vi "GetGreyscalePlane.vi"(1 "Image In":T1 {"Dialogs" format="%.0b"}) -> (0 "Greyscale  Out":T1 {"Dialogs" format="%.0b"})   [LabVIEW 2024]
uses:
  <userlib>/ImageProcessing/QTLIB_2595_LV86/QT_Image.ctl
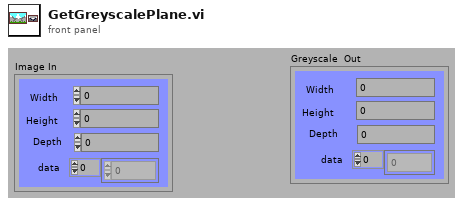
[diagram p1: front panel]
types:
  T1 = typedef "QT_Image.ctl" = cluster{"Width":i32, "Height":i32, "Depth":i32, "data":u8[], "Compressed data":u8[], "Color table":u32[], "Duration":i32, "Options":i32, "Timestamp":i32, "ID":i32, "Reserved":i32, "Dialogs":u32}
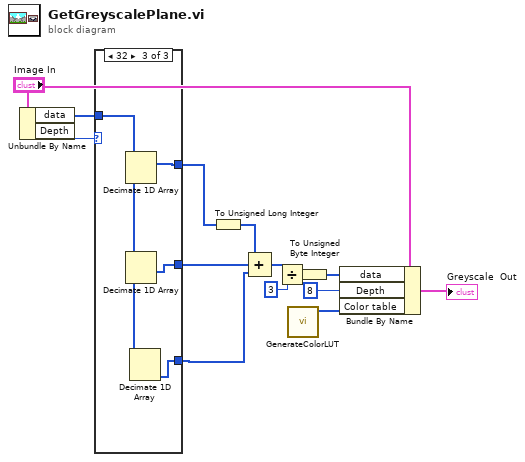
[diagram p0: block diagram]
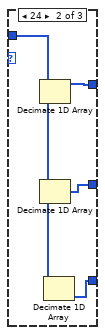
[diagram p3: hidden frame]
diagram:
  n1 = Unbundle By Name("Image In") -> ("data"=w14:u8[], "Depth"=w13:i32)
  n2 = case shown="32" w13 {
    tunnel: [w15 w17 w21] -> w12
    tunnel: w14 -> [w15 w19 w23]
    tunnel: [w15 w18 w22] -> w11
    tunnel: [w15 w16 w20] -> w10
    frame Default {
    }
    frame 24 {
      n3 = Decimate 1D Array(w19) -> (w17:u8[])  [unwired: 2 out]
      n4 = Decimate 1D Array(w19) -> (w18:u8[])  [unwired: 2 out]
      n5 = Decimate 1D Array(w19) -> (w16:u8[])  [unwired: 2 out]
    }
    frame 32 {
      n6 = Decimate 1D Array(w23) -> (w21:u8[])  [unwired: 3 out]
      n7 = Decimate 1D Array(w23) -> (w22:u8[])  [unwired: 3 out]
      n8 = Decimate 1D Array(w23) -> (w20:u8[])  [unwired: 3 out]
    }
  }
  n9 = To Unsigned Long Integer(number=w12) -> (unsigned 32bit integer=w9:u32[])
  n10 = Compound Arithmetic op=ADD(w9, w11, w10) -> (w8:u32[])
  n11 = Divide(x=w8, y=3 ("Depth")) -> (x/y=w5:dbl[])
  n12 = call <userlib>:"GenerateColorLUT.vi"() -> ("Greyscale"=w2:u32[])  [unwired: 4 out]
  n13 = To Unsigned Byte Integer(number=w5) -> (unsigned 8bit integer=w1:u8[])
  n14 = Bundle By Name(cluster="Image In", "data"=w1, "Depth"=8, "Color table"=w2) -> (→"Greyscale  Out":T1)
